vi "Hue_Color_value.vi"(1 "Hue":dbl) -> (0 "Color":T1)   [LabVIEW 2019]
uses:
  Implements/Control_Panel/TypeDefs/ControlPanelColor.ctl
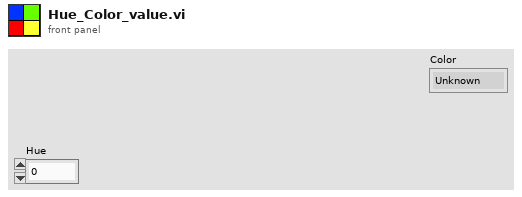
[diagram p1: front panel]
types:
  T1 = typedef "ControlPanelColor.ctl" = enum16{"Unknown", "Red", "Green", "Blue", "Yellow"}
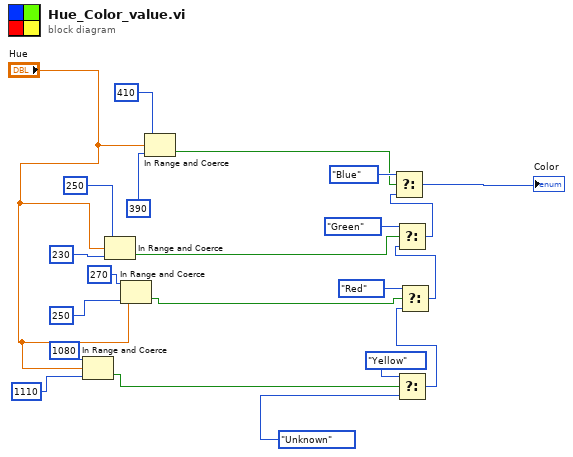
[diagram p0: block diagram]
diagram:
  n1 = In Range and Coerce(upper limit=1080, x="Hue", lower limit=1110) -> (In Range?=w2:bool)  [unwired: 1 out]
  n2 = In Range and Coerce(upper limit=250, x="Hue", lower limit=230) -> (In Range?=w9:bool)  [unwired: 1 out]
  n3 = In Range and Coerce(upper limit=270, x="Hue", lower limit=250) -> (In Range?=w6:bool)  [unwired: 1 out]
  n4 = In Range and Coerce(upper limit=410, x="Hue", lower limit=390) -> (In Range?=w12:bool)  [unwired: 1 out]
  n5 = Select(t=ControlPanelColor."Yellow", s=w2, f=ControlPanelColor."Unknown" ("Color 2")) -> (s? t:f=w19:T1)
  n6 = Select(t=ControlPanelColor."Red", s=w6, f=w19) -> (s? t:f=w18:T1)
  n7 = Select(t=ControlPanelColor."Green", s=w9, f=w18) -> (s? t:f=w17:T1)
  n8 = Select(t=ControlPanelColor."Blue", s=w12, f=w17) -> (s? t:f=→"Color":T1)
